vi "GV buffer-in ready.vi"() -> ()   [LabVIEW 2017]
panel:
  in  "Buffer-in ready":bool
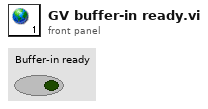
[diagram p1: front panel]
diagram:
